vi "TestWithPowerReads.vi"() -> ()   [LabVIEW 2012]
panel:
  in  "stop":bool
  out "concatenated string":string
  out "Original Register Map":string
  out "Register Map":string
  out "UDP Close Error":errorcluster
  in  "port":u16=300
  out "UDP Open Error":errorcluster
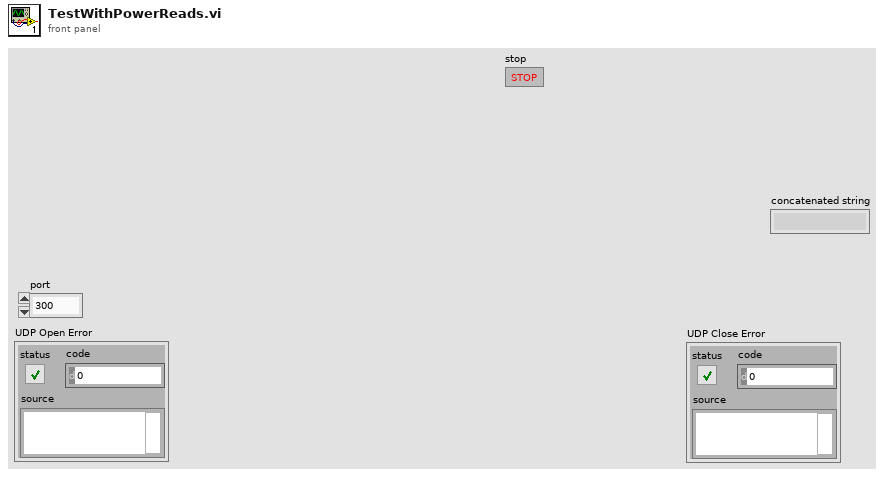
[diagram p1: front panel]
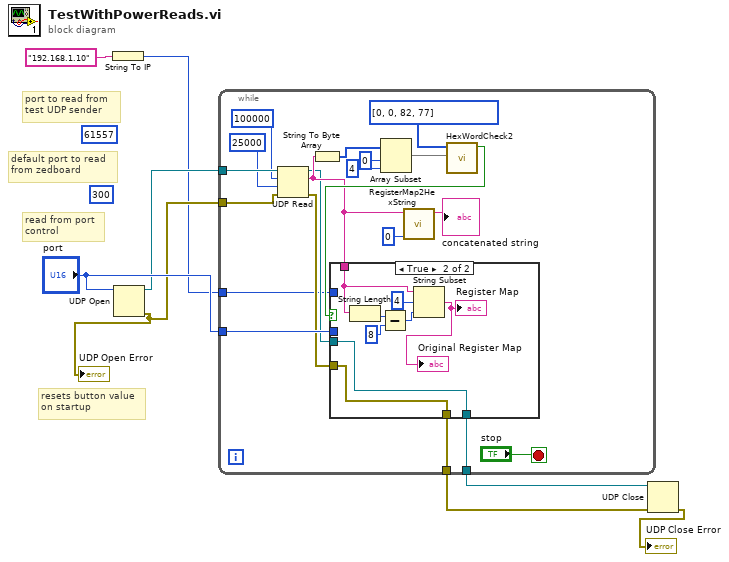
[diagram p0: block diagram]
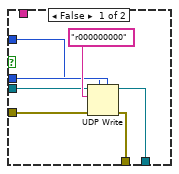
[diagram p2: hidden frame]
diagram:
  (unwired) u16 300 ("port")
  (unwired) u16 61557 ("port")
  # "resets button value \non startup"
  # "default port to read \nfrom zedboard"
  # "read from port\ncontrol"
  # "port to read from \ntest UDP sender"
  n1 = String To IP(1:"192.168.1.10" ("name")) -> (0:w1:u32)
  n2 = UDP Open(11:"port") -> (port=w2:refnum<k16>, 0:w3:errorcluster)  [unwired: 4 in, 1 out]
  "UDP Open Error" <- w3
  n3 = while {
    tunnel: w3 -> [w28]
    tunnel: w2 -> [w27]
    tunnel: [w11] -> w6
    tunnel: "port" -> [w15]
    tunnel: [w13] -> w4
    tunnel: w1 -> [w10]
    stop <- "stop" stop-if-true
    n4 = UDP Read(connection ID=w27, max size (548)=100000, timeout ms (25000)=25000, 8:w28) -> (data out=w18:string, error out=w14:errorcluster, 3:w12:refnum<k16>)  [unwired: 2 out]
    n5 = String To Byte Array(string=w18) -> (unsigned byte array=w22:u8[])
    n6 = Array Subset(array=w22, index=0, length=4) -> (w21:u8[])
    n7 = call "RegisterMap2HexString.vi"("Word Num"=0, "string"=w18) -> ("concatenated string"=→"concatenated string":string)  [unwired: 9 in]
    n8 = call "HexWordCheck2.vi"("array"=w21, "Input Array"=u8[] [0, 0, 82, 77]) -> ("Boolean"=w23:bool)  [unwired: 9 in]
    n9 = case shown="True" w23 {
      tunnel: w18 -> [_ w39]
      tunnel: w15 -> [w34 _]
      tunnel: w14 -> [w33 w37]
      tunnel: [w32 w37] -> w13
      tunnel: w12 -> [w31 w36]
      tunnel: [w30 w36] -> w11
      tunnel: w10 -> [w29 _]
      frame False {
        n10 = UDP Write(address=w29, port or service name=w34, connection ID=w31, data in="r000000000", 8:w33) -> (error out=w32:errorcluster, 3:w30:refnum<k16>)  [unwired: 1 in]
      }
      frame True {
        n11 = String Length(string=w39) -> (length=w41:i32)
        n12 = Subtract(x=w41, y=8) -> (x-y=w43:i32)
        n13 = String Subset(string=w39, offset (0)=4, length (rest)=w43) -> (substring=→"Register Map" →"Original Register Map":string)
      }
    }
  }
  n14 = UDP Close(connection ID=w6, 8:w4) -> (error out=→"UDP Close Error":errorcluster)  [unwired: 1 out]
